vi "adapt_range.vi"(8 "error in (no error)":errorcluster, 9 "range old":cluster{dbl, dbl}(slide)={255.0, 255.0} scale=0.0..1.0, 10 "range new":cluster{dbl, dbl}(slide)={255.0, 255.0} scale=0.0..1.0, 11 "ColorOverlay in":refnum<class "ColorOverlay.lvclass">) -> (0 "error out":errorcluster, 3 "ColorOverlay out":refnum<class "ColorOverlay.lvclass">)   [LabVIEW 2010, in "ColorOverlay.lvclass"]
uses:
  ColorOverlay.lvclass
  ColorOverlay.lvclass/ColorOverlay.ctl
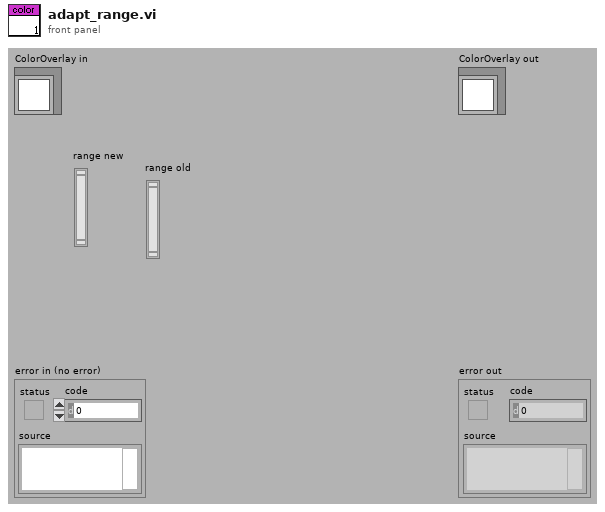
[diagram p1: front panel]
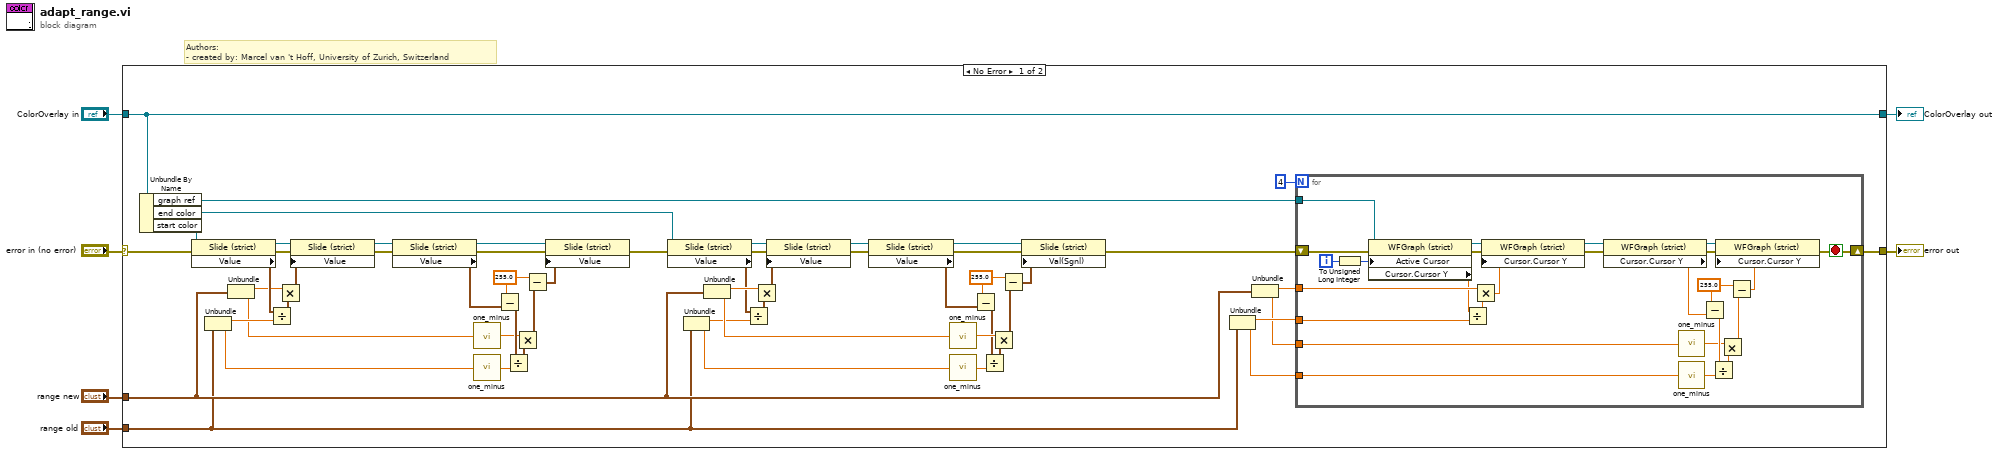
[diagram p0: block diagram]
diagram:
  # "Authors: \n- created by: Marcel van 't Hoff, University of Zurich, Switzerland"
  n1 = case shown="No Error" "error in (no error)" {
    selector: "error in (no error)" -> [w56 w91]
    tunnel: [w37 w91] -> w5
    tunnel: [w63 w90] -> w3
    tunnel: "ColorOverlay in" -> [w63 w90]
    tunnel: "range new" -> [w12 _]
    tunnel: "range old" -> [w11 _]
    frame No Error {
      w36 = 255.0 ("x")
      w38 = 255.0 ("x")
      n2 = Unbundle By Name(w63) -> ("graph ref"=w55:refnum<vi>, "end color"=w15:refnum<vi>, "start color"=w62:refnum<vi>)
      n3 = property class="Slide (strict)"(reference=w62, error in=w56) -> (reference out=w61:refnum<vi>, error out=w60:errorcluster, "Value"=w59:cluster{dbl, dbl, dbl, dbl})
      n4 = Unbundle(w11) -> (w49:dbl, w42:dbl)
      n5 = Unbundle(w12) -> (w50:dbl, w41:dbl)
      n6 = Divide(x=w59, y=w49) -> (x/y=w58:cluster{dbl, dbl, dbl, dbl})
      n7 = Multiply(x=w50, y=w58) -> (x*y=w57:cluster{dbl, dbl, dbl, dbl})
      n8 = property class="Slide (strict)"(reference=w61, error in=w60, "Value"=w57) -> (reference out=w43:refnum<vi>, error out=w44:errorcluster)
      n9 = property class="Slide (strict)"(reference=w43, error in=w44) -> (reference out=w52:refnum<vi>, error out=w53:errorcluster, "Value"=w48:cluster{dbl, dbl, dbl, dbl})
      n10 = call "one_minus.vi"("x"=w41) -> ("1-x"=w40:dbl)  [unwired: 4 in]
      n11 = call "one_minus.vi"("x"=w42) -> ("1-x"=w39:dbl)  [unwired: 4 in]
      n12 = Subtract(x=w38, y=w48) -> (x-y=w47:cluster{dbl, dbl, dbl, dbl})
      n13 = Divide(x=w47, y=w39) -> (x/y=w51:cluster{dbl, dbl, dbl, dbl})
      n14 = Multiply(x=w40, y=w51) -> (x*y=w46:cluster{dbl, dbl, dbl, dbl})
      n15 = Subtract(x=w38, y=w46) -> (x-y=w45:cluster{dbl, dbl, dbl, dbl})
      n16 = property class="Slide (strict)"(reference=w52, error in=w53, "Value"=w45) -> (error out=w14:errorcluster)  [unwired: 1 out]
      n17 = property class="Slide (strict)"(reference=w15, error in=w14) -> (reference out=w16:refnum<vi>, error out=w17:errorcluster, "Value"=w18:cluster{dbl, dbl, dbl, dbl})
      n18 = Unbundle(w11) -> (w25:dbl, w32:dbl)
      n19 = Unbundle(w12) -> (w24:dbl, w33:dbl)
      n20 = Divide(x=w18, y=w25) -> (x/y=w19:cluster{dbl, dbl, dbl, dbl})
      n21 = Multiply(x=w24, y=w19) -> (x*y=w20:cluster{dbl, dbl, dbl, dbl})
      n22 = property class="Slide (strict)"(reference=w16, error in=w17, "Value"=w20) -> (reference out=w31:refnum<vi>, error out=w30:errorcluster)
      n23 = property class="Slide (strict)"(reference=w31, error in=w30) -> (reference out=w22:refnum<vi>, error out=w21:errorcluster, "Value"=w26:cluster{dbl, dbl, dbl, dbl})
      n24 = call "one_minus.vi"("x"=w33) -> ("1-x"=w34:dbl)  [unwired: 4 in]
      n25 = call "one_minus.vi"("x"=w32) -> ("1-x"=w35:dbl)  [unwired: 4 in]
      n26 = Subtract(x=w36, y=w26) -> (x-y=w27:cluster{dbl, dbl, dbl, dbl})
      n27 = Divide(x=w27, y=w35) -> (x/y=w23:cluster{dbl, dbl, dbl, dbl})
      n28 = Multiply(x=w34, y=w23) -> (x*y=w28:cluster{dbl, dbl, dbl, dbl})
      n29 = Subtract(x=w36, y=w28) -> (x-y=w29:cluster{dbl, dbl, dbl, dbl})
      n30 = property class="Slide (strict)"(reference=w22, error in=w21, "Val(Sgnl)"=w29) -> (error out=w13:errorcluster)  [unwired: 1 out]
      n31 = Unbundle(w11) -> (w9:dbl, w7:dbl)
      n32 = Unbundle(w12) -> (w10:dbl, w8:dbl)
      n33 = for {
        N: 4 -> [_]
        tunnel: w55 -> [w89]
        shift-right: [w74] -> w37
        shift-left: w13 -> [w88]
        tunnel: w10 -> [w82]
        tunnel: w9 -> [w81]
        tunnel: w8 -> [w67]
        tunnel: w7 -> [w66]
        i -> [w85]
        stop <- w74 stop-if-true
        w68 = 255.0 ("x")
        n34 = To Unsigned Long Integer(number=w85) -> (unsigned 32bit integer=w84:u32)
        n35 = property class="WFGraph (strict)"(reference=w89, error in=w88, "Active Cursor"=w84) -> (reference out=w86:refnum<vi>, error out=w87:errorcluster, "Cursor.Cursor Y"=w80:dbl)
        n36 = Divide(x=w80, y=w81) -> (x/y=w83:dbl)
        n37 = Multiply(x=w82, y=w83) -> (x*y=w79:dbl)
        n38 = property class="WFGraph (strict)"(reference=w86, error in=w87, "Cursor.Cursor Y"=w79) -> (reference out=w77:refnum<vi>, error out=w76:errorcluster)
        n39 = property class="WFGraph (strict)"(reference=w77, error in=w76) -> (reference out=w78:refnum<vi>, error out=w75:errorcluster, "Cursor.Cursor Y"=w65:dbl)
        n40 = call "one_minus.vi"("x"=w67) -> ("1-x"=w70:dbl)  [unwired: 4 in]
        n41 = call "one_minus.vi"("x"=w66) -> ("1-x"=w69:dbl)  [unwired: 4 in]
        n42 = Subtract(x=w68, y=w65) -> (x-y=w72:dbl)
        n43 = Divide(x=w72, y=w69) -> (x/y=w73:dbl)
        n44 = Multiply(x=w70, y=w73) -> (x*y=w71:dbl)
        n45 = Subtract(x=w68, y=w71) -> (x-y=w64:dbl)
        n46 = property class="WFGraph (strict)"(reference=w78, error in=w75, "Cursor.Cursor Y"=w64) -> (error out=w74:errorcluster)  [unwired: 1 out]
      }
    }
    frame Error {
    }
  }
  "error out" <- w5
  "ColorOverlay out" <- w3
